vi "Add Index (DNet Output Bytes).vi"(8 "Count":i32, 9 "Enabled":bool, 10 "Byte":u8, 11 "Indices Input":i32[](array[numeric])) -> (0 "Count+1":i32, 3 "Indices Output":i32[](array[numeric]))   [LabVIEW 2011]
uses:
  GlobalVariables.vi
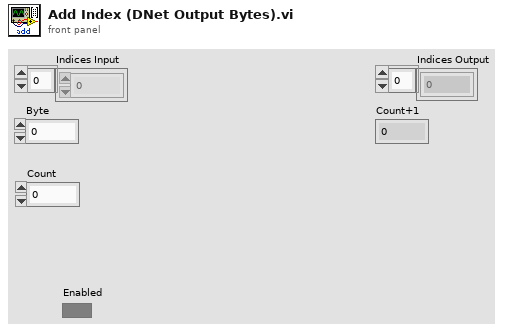
[diagram p1: front panel]
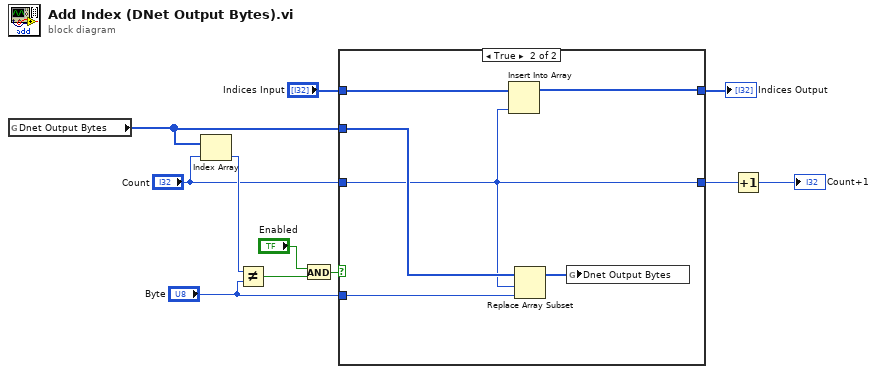
[diagram p0: block diagram]
diagram:
  n1 = global read "GlobalVariables.vi" "Dnet Output Bytes"() -> (w11:u8[])
  n2 = Index Array(array=w11, index="Count") -> (element=w10:u8)
  n3 = Not Equal?(x=w10, y="Byte") -> (x != y?=w2:bool)
  n4 = And(x="Enabled", y=w2) -> (x .and. y?=w1:bool)
  n5 = case shown="True" w1 {
    tunnel: w11 -> [_ w18]
    tunnel: "Indices Input" -> [w13 w17]
    tunnel: [w13 w16] -> w8
    tunnel: "Byte" -> [_ w15]
    tunnel: "Count" -> [w12 w14]
    tunnel: [w12 w14] -> w5
    frame False {
    }
    frame True {
      n6 = Insert Into Array(array=w17, new element=w14) -> (w16:i32[])  [unwired: 1 in]
      n7 = Replace Array Subset(array=w18, new element=w15, index=w14) -> (w19:u8[])
      n8 = global write "GlobalVariables.vi" "Dnet Output Bytes"(w19) -> ()
    }
  }
  "Indices Output" <- w8
  n9 = Increment(x=w5) -> (x+1=→"Count+1":i32)
